vi "Initialize Thermocouples.vi"(8 "error in":errorcluster, 9 "Sensor sample period (ms)":i32=100, 11 "file path":path) -> (0 "Error Out":errorcluster, 3 "task out":refnum<k21>)   [LabVIEW 2018]
uses:
  <vilib>/DAQmx/create/channels.llb/DAQmx Create Channel (AI-Temperature-Thermocouple).vi
  <vilib>/DAQmx/configure/timing.llb/DAQmx Timing (Sample Clock).vi
  <vilib>/DAQmx/configure/task.llb/DAQmx Configure Logging (TDMS).vi
  <resource>/objmgr/daqmx.rc
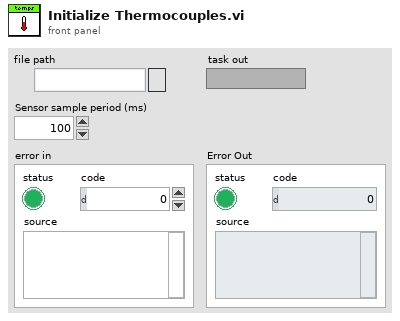
[diagram p1: front panel]
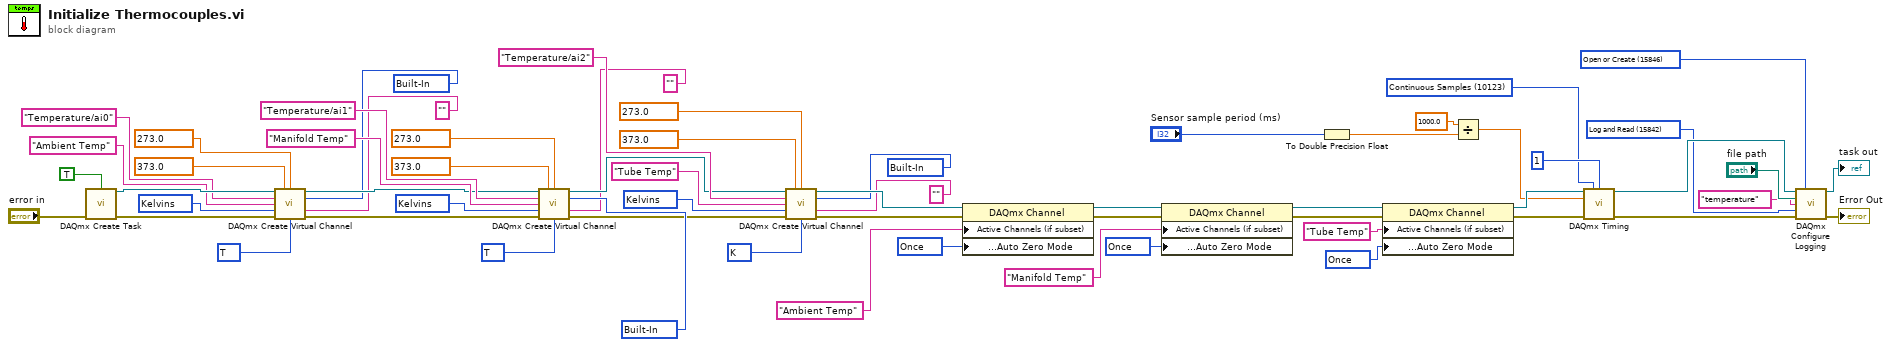
[diagram p0: block diagram]
diagram:
  w6 = 15846 items=["Open"=10437, "Open or Create"=15846, "Create or Replace"=15847, "Create"=15848] ("operation")
  w7 = 15842 items=["Off"=10231, "Log"=15844, "Log and Read"=15842] ("logging mode")
  w15 = 10123 items=["Finite Samples"=10178, "Continuous Samples"=10123, "Hardware Timed Single Point"=12522] ("sample mode")
  w54 = 10244 items=["None"=10230, "Once"=10244, "Every Sample"=10164] ("AutoZeroMode")
  w50 = 10244 items=["None"=10230, "Once"=10244, "Every Sample"=10164] ("AutoZeroMode")
  w46 = 10244 items=["None"=10230, "Once"=10244, "Every Sample"=10164] ("AutoZeroMode")
  w45 = 10200 items=["Built-In"=10200, "Constant Value"=10116, "Channel"=10113] ("cjc source")
  w42 = 10073 items=["J"=10072, "K"=10073, "N"=10077, "R"=10082, "S"=10085, "T"=10086, "B"=10047, "E"=10055] ("thermocouple type")
  w41 = 10325 items=["deg C"=10143, "deg F"=10144, "Kelvins"=10325, "deg R"=10145, "From Custom Scale"=10065] ("units")
  w35 = 10200 items=["Built-In"=10200, "Constant Value"=10116, "Channel"=10113] ("cjc source")
  w32 = 10086 items=["J"=10072, "K"=10073, "N"=10077, "R"=10082, "S"=10085, "T"=10086, "B"=10047, "E"=10055] ("thermocouple type")
  w31 = 10325 items=["deg C"=10143, "deg F"=10144, "Kelvins"=10325, "deg R"=10145, "From Custom Scale"=10065] ("units")
  w25 = 10200 items=["Built-In"=10200, "Constant Value"=10116, "Channel"=10113] ("cjc source")
  w22 = 10086 items=["J"=10072, "K"=10073, "N"=10077, "R"=10082, "S"=10085, "T"=10086, "B"=10047, "E"=10055] ("thermocouple type")
  w21 = 10325 items=["deg C"=10143, "deg F"=10144, "Kelvins"=10325, "deg R"=10145, "From Custom Scale"=10065] ("units")
  n1 = call <vilib>:"DAQmx Create Task.vi"("auto cleanup"=TRUE, "error in"="error in") -> ("task out"=w58:refnum<k21>, "error out"=w57:errorcluster)  [unwired: 12 in]
  n2 = call-poly <vilib>:"DAQmx Create Virtual Channel.vi"("task in"=w58, "maximum value"=373.0, "minimum value"=273.0, "physical channels"="Temperature/ai0" ("physical channel"), "cjc source"=w25, "name to assign"="Ambient Temp" ("channel name"), "units"=w21, "cjc channel"="", "error in"=w57, "thermocouple type"=w22) -> ("task out"=w26:refnum<k21>, "error out"=w20:errorcluster)  [unwired: 4 in]
  n3 = call-poly <vilib>:"DAQmx Create Virtual Channel.vi"("task in"=w26, "maximum value"=373.0, "minimum value"=273.0, "physical channels"="Temperature/ai1" ("physical channel"), "cjc source"=w35, "name to assign"="Manifold Temp" ("channel name"), "units"=w31, "cjc channel"="", "error in"=w20, "thermocouple type"=w32) -> ("task out"=w36:refnum<k21>, "error out"=w30:errorcluster)  [unwired: 4 in]
  n4 = call-poly <vilib>:"DAQmx Create Virtual Channel.vi"("task in"=w36, "maximum value"=373.0, "minimum value"=273.0, "physical channels"="Temperature/ai2" ("physical channel"), "cjc source"=w45, "name to assign"="Tube Temp" ("channel name"), "units"=w41, "cjc channel"="", "error in"=w30, "thermocouple type"=w42) -> ("task out"=w48:refnum<k21>, "error out"=w40:errorcluster)  [unwired: 4 in]
  n5 = property on="Property Node" class="DAQmx Channel"(reference=w48, error in=w40, "Active Channels (if subset)"="Ambient Temp" ("ActiveChan"), "Analog Input:General Properties:Advanced:High Accuracy Settings:Auto Zero Mode"=w46) -> (reference out=w52:refnum<k21>, error out=w49:errorcluster)
  n6 = property on="Property Node" class="DAQmx Channel"(reference=w52, error in=w49, "Active Channels (if subset)"="Manifold Temp" ("ActiveChan"), "Analog Input:General Properties:Advanced:High Accuracy Settings:Auto Zero Mode"=w50) -> (reference out=w56:refnum<k21>, error out=w53:errorcluster)
  n7 = To Double Precision Float(number="Sensor sample period (ms)") -> (double precision float=w3:dbl)
  n8 = property on="Property Node" class="DAQmx Channel"(reference=w56, error in=w53, "Active Channels (if subset)"="Tube Temp" ("ActiveChan"), "Analog Input:General Properties:Advanced:High Accuracy Settings:Auto Zero Mode"=w54) -> (reference out=w13:refnum<k21>, error out=w14:errorcluster)
  n9 = Divide(x=1000.0, y=w3) -> (x/y=w1:dbl)
  n10 = call-poly <vilib>:"DAQmx Timing.vi"("task/channels in"=w13, "sample mode"=w15, "samples per channel"=1 ("number of samples"), "rate"=w1, "error in"=w14) -> ("task out"=w11:refnum<k21>, "error out"=w10:errorcluster)  [unwired: 9 in]
  n11 = call-poly <vilib>:"DAQmx Configure Logging.vi"("task/channels in"=w11, "operation"=w6, "file path"="file path", "group name"="temperature", "logging mode"=w7, "error in"=w10) -> ("task out"=→"task out":refnum<k21>, "error out"=→"Error Out":errorcluster)  [unwired: 8 in]
